vi "dfd_Neg Real & Pos Imag.vi"(1 "complex in":cdb format="%.2f") -> (0 "complex out":cdb format="%.2f")   [LabVIEW 2017, in "NI_DigFilter_Design.lvlib"]
uses:
  <vilib>/addons/Digital Filter Design/NI_DigFilter_Design.lvlib
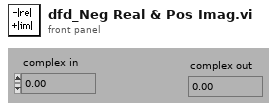
[diagram p1: front panel]
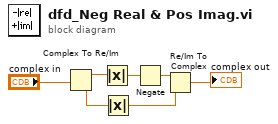
[diagram p0: block diagram]
diagram:
  n1 = Complex To Re/Im(x + iy="complex in") -> (x=w6:dbl, y=w5:dbl)
  n2 = Absolute Value(x=w6) -> (abs(x)=w4:dbl)
  n3 = Absolute Value(x=w5) -> (abs(x)=w2:dbl)
  n4 = Negate(x=w4) -> (-x=w3:dbl)
  n5 = Re/Im To Complex(1:w2, 2:w3) -> (0:→"complex out":cdb)
